vi "Build All.vi"() -> ()   [LabVIEW 2021]
uses:
  <vilib>/CIF Foundation/CIF LabVIEW Scripting/LV Scripting/Typedef/Version Increment.ctl
  <vilib>/CIF Foundation/CIF LabVIEW Scripting/LV Scripting/Typedef/Version.ctl
  <vilib>/CIF Foundation/CIF Core/CIFUtilities/Scripting/Build Libraries/LabVIEW Build Script/LabVIEW Build Script.lvclass/LabVIEW Build Script.ctl
  <vilib>/CIF Foundation/CIF LabVIEW Scripting/LV Scripting/SubVIs/Add Scripting Error.vi
  <vilib>/CIF Foundation/CIF Utilities/Errors/Append Error Location.vi
  <vilib>/AppBuilder/AB_API_Simple/Build (path).vi
  <vilib>/AppBuilder/AB_API_Simple/NI_App_Builder_API.lvlib
  <vilib>/CIF Foundation/CIF LabVIEW Scripting/LV Scripting/LV Scripting Utilities.lvlib
  <vilib>/CIF Foundation/CIF Core/CIFUtilities/Scripting/Build Libraries/LabVIEW Build Script/LabVIEW Build Script.lvclass
panel:
  out "error out 3":errorcluster
  out "error out 2":errorcluster
  out "Version":T1
  in  "String":string
  in  "Changes":string
  in  "Version Increment":T2
  out "error out":errorcluster
  out "Description":string
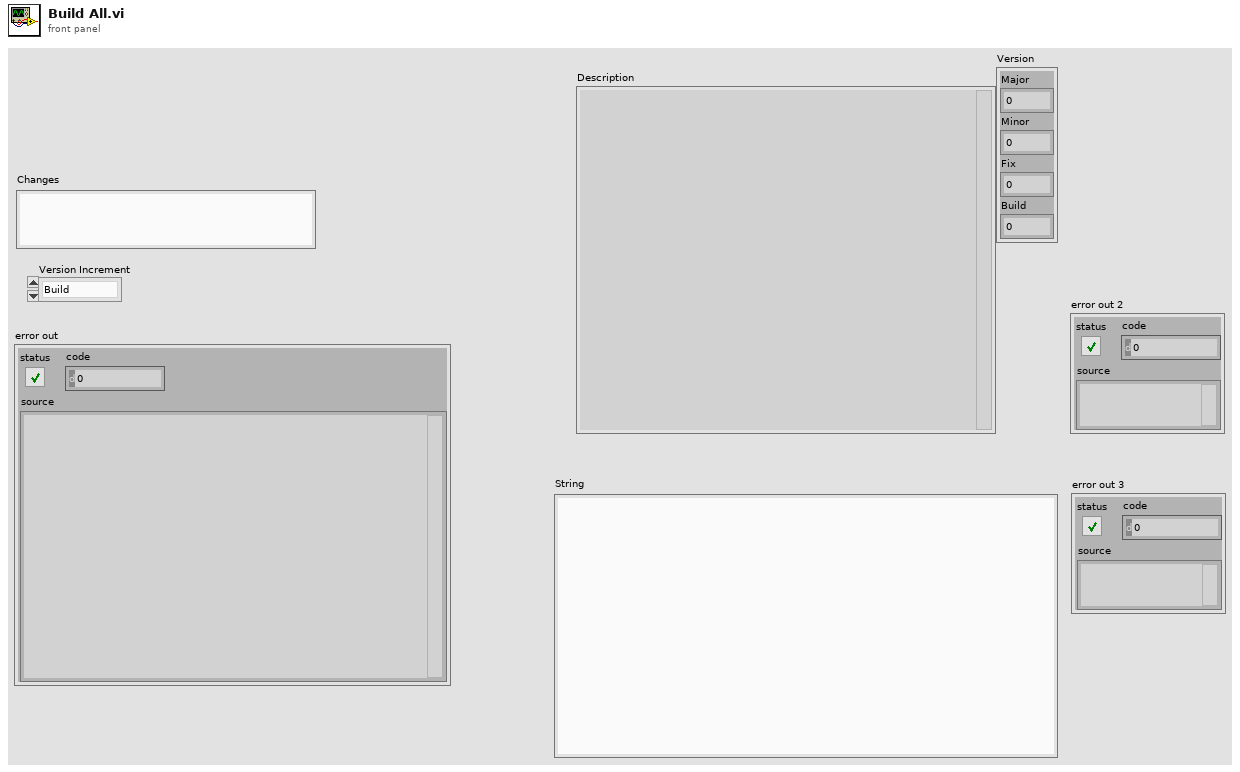
[diagram p1: front panel]
types:
  T1 = typedef "Version.ctl" = cluster{"Major":u16, "Minor":u16, "Fix":u16, "Build":u16}
  T2 = typedef "LV Scripting Utilities.lvlib/Version Increment.ctl" = enum16{"Build", "Fix", "Minor", "Major"}
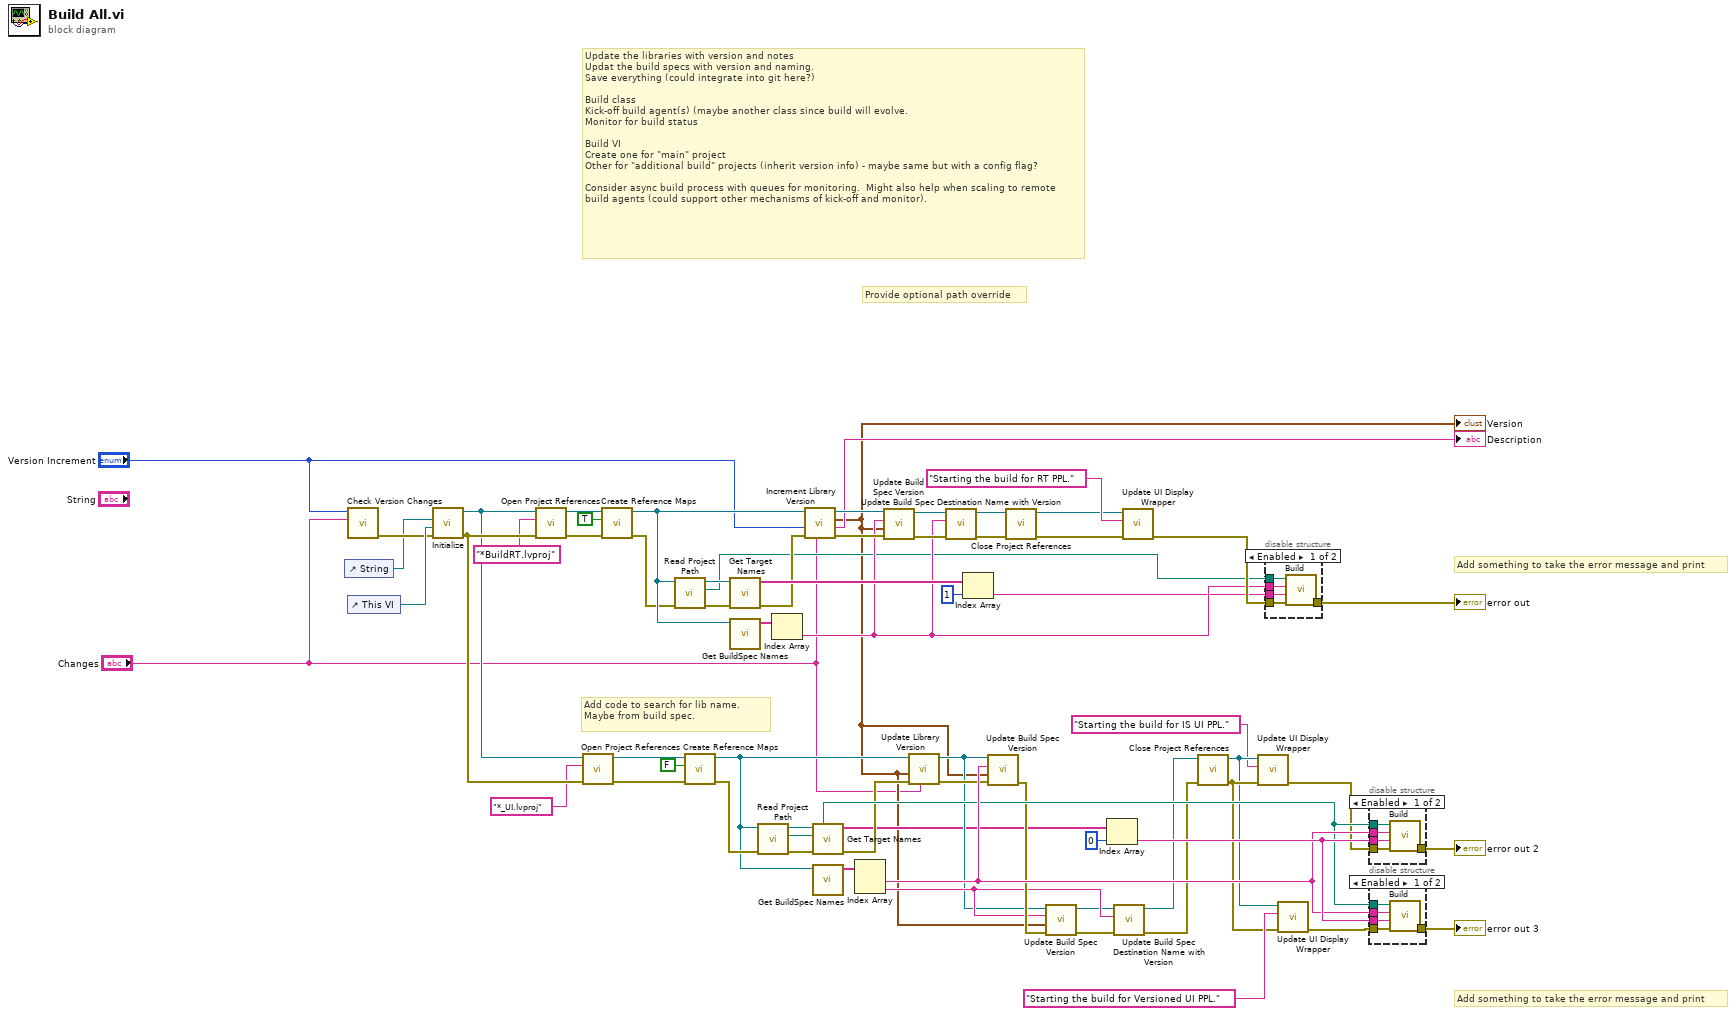
[diagram p0: block diagram]
diagram:
  # "Add code to search for lib name. Maybe from build spec."
  # "Add something to take the error message and print"
  # "Add something to take the error message and print"
  # "Update the libraries with version and notes\nUpdat the build specs with version and naming.\nSave everything (could integrate into git here?)\n\nBuild class\nKick-off build agent(s) (maybe another class since build will evolve.\nMonitor for build status\n\nBuild VI\nCreate one for \"main\" project\nOther for \"additional build\" projects (inherit version info) - maybe same but with a config flag?\n\nConsider async build process with queues for monitoring.  Might also help when scaling to remote build agents (could support other mechanisms of kick-off and monitor)."
  # "Provide optional path override"
  n1 = control-ref of="String"() -> (w12:refnum<vi>)
  n2 = call <vilib>:"Check Version Changes.vi"("Changes"="Changes", "Version Increment"="Version Increment") -> ("error out"=w17:errorcluster)  [unwired: 9 in]
  n3 = control-ref of="This VI"() -> (w24:refnum<vi>)
  n4 = call <vilib>:"Initialize.vi"("error in (no error)"=w17, "Calling VI"=w24, "UI Display"=w12) -> ("error out"=w38:errorcluster, "LabVIEW Build Script out"=w36:refnum<class "LabVIEW Build Script.lvclass">)  [unwired: 7 in]
  n5 = call <vilib>:"Open Project References.vi"("error in (no error)"=w38, "Search Pattern"="*BuildRT.lvproj" ("pattern"), "LabVIEW Build Script in"=w36) -> ("error out"=w15:errorcluster, "LabVIEW Build Script out"=w14:refnum<class "LabVIEW Build Script.lvclass">)  [unwired: 7 in]
  n6 = call <vilib>:"Open Project References.vi"("error in (no error)"=w38, "Search Pattern"="*_UI.lvproj" ("pattern"), "LabVIEW Build Script in"=w36) -> ("error out"=w50:errorcluster, "LabVIEW Build Script out"=w49:refnum<class "LabVIEW Build Script.lvclass">)  [unwired: 7 in]
  n7 = call <vilib>:"Create Reference Maps.vi"("error in (no error)"=w15, "RT Target"=TRUE, "LabVIEW Build Script in"=w14) -> ("error out"=w29:errorcluster, "LabVIEW Build Script out"=w30:refnum<class "LabVIEW Build Script.lvclass">)  [unwired: 7 in]
  n8 = call <vilib>:"Read Project Path.vi"("error in (no error)"=w29, "LabVIEW Build Script in"=w30) -> ("error out"=w31:errorcluster, "Project Path"=w8:path, "LabVIEW Build Script out"=w32:refnum<class "LabVIEW Build Script.lvclass">)  [unwired: 7 in]
  n9 = call <vilib>:"Create Reference Maps.vi"("error in (no error)"=w50, "RT Target"=FALSE, "LabVIEW Build Script in"=w49) -> ("error out"=w42:errorcluster, "LabVIEW Build Script out"=w41:refnum<class "LabVIEW Build Script.lvclass">)  [unwired: 7 in]
  n10 = call <vilib>:"Get Target Names.vi"("error in (no error)"=w31, "LabVIEW Build Script in"=w32) -> ("error out"=w25:errorcluster, "Project Targets"=w27:string[])  [unwired: 8 in]
  n11 = call <vilib>:"Get BuildSpec Names.vi"("LabVIEW Build Script in"=w30) -> ("BuildSpecs"=w26:string[])  [unwired: 10 in]
  n12 = call <vilib>:"Read Project Path.vi"("error in (no error)"=w42, "LabVIEW Build Script in"=w41) -> ("error out"=w40:errorcluster, "Project Path"=w64:path, "LabVIEW Build Script out"=w39:refnum<class "LabVIEW Build Script.lvclass">)  [unwired: 7 in]
  n13 = Index Array(array=w26) -> (element=w10:string)  [unwired: 1 in]
  n14 = call <vilib>:"Increment Library Version.vi"("Changes"="Changes", "error in (no error)"=w25, "Version Increment"="Version Increment", "LabVIEW Build Script in"=w30) -> ("error out"=w19:errorcluster, "Description"=→"Description":string, "Version"=w3:T1, "LabVIEW Build Script out"=w18:refnum<class "LabVIEW Build Script.lvclass">)  [unwired: 4 in]
  "Version" <- w3
  n15 = call <vilib>:"Get Target Names.vi"("error in (no error)"=w40, "LabVIEW Build Script in"=w39) -> ("error out"=w46:errorcluster, "Project Targets"=w44:string[])  [unwired: 8 in]
  n16 = call <vilib>:"Get BuildSpec Names.vi"("LabVIEW Build Script in"=w41) -> ("BuildSpecs"=w45:string[])  [unwired: 10 in]
  n17 = Index Array(array=w45) -> (element #1=w65:string, element #2=w55:string)  [unwired: 2 in]
  n18 = call <vilib>:"Update Build Spec Version.vi"("error in (no error)"=w19, "Version"=w3, "Search Pattern"=w10, "LabVIEW Build Script in"=w18) -> ("error out"=w21:errorcluster, "LabVIEW Build Script out"=w20:refnum<class "LabVIEW Build Script.lvclass">)  [unwired: 6 in]
  n19 = call <vilib>:"Update Library Version.vi"("Changes"="Changes", "error in (no error)"=w46, "Version"=w3, "LabVIEW Build Script in"=w41) -> ("error out"=w53:errorcluster, "LabVIEW Build Script out"=w52:refnum<class "LabVIEW Build Script.lvclass">)  [unwired: 5 in, 1 out]
  n20 = call <vilib>:"Update Build Spec Destination Name with Version.vi"("error in (no error)"=w21, "Search Pattern"=w10, "LabVIEW Build Script in"=w20) -> ("error out"=w23:errorcluster, "LabVIEW Build Script out"=w22:refnum<class "LabVIEW Build Script.lvclass">)  [unwired: 7 in]
  n21 = Index Array(array=w27, index=1) -> (element=w9:string)
  n22 = call <vilib>:"Update Build Spec Version.vi"("error in (no error)"=w53, "Version"=w3, "Search Pattern"=w65, "LabVIEW Build Script in"=w52) -> ("error out"=w56:errorcluster)  [unwired: 6 in, 1 out]
  n23 = call <vilib>:"Close Project References.vi"("error in (no error)"=w23, "LabVIEW Build Script in"=w22) -> ("error out"=w34:errorcluster, "LabVIEW Build Script out"=w33:refnum<class "LabVIEW Build Script.lvclass">)  [unwired: 8 in]
  n24 = call <vilib>:"Update Build Spec Version.vi"("error in (no error)"=w56, "Version"=w3, "Search Pattern"=w55, "LabVIEW Build Script in"=w52) -> ("error out"=w54:errorcluster, "LabVIEW Build Script out"=w51:refnum<class "LabVIEW Build Script.lvclass">)  [unwired: 6 in]
  n25 = Index Array(array=w44, index=0) -> (element=w66:string)
  n26 = call <vilib>:"Update Build Spec Destination Name with Version.vi"("error in (no error)"=w54, "Search Pattern"=w55, "LabVIEW Build Script in"=w51) -> ("error out"=w58:errorcluster, "LabVIEW Build Script out"=w57:refnum<class "LabVIEW Build Script.lvclass">)  [unwired: 7 in]
  n27 = call <vilib>:"Update UI Display Wrapper.vi"("error in (no error)"=w34, "Update for Display"="Starting the build for RT PPL.", "LabVIEW Build Script in"=w33) -> ("error out"=w11:errorcluster)  [unwired: 8 in]
  n28 = call <vilib>:"Close Project References.vi"("error in (no error)"=w58, "LabVIEW Build Script in"=w57) -> ("error out"=w61:errorcluster, "LabVIEW Build Script out"=w60:refnum<class "LabVIEW Build Script.lvclass">)  [unwired: 8 in]
  n29 = call <vilib>:"Update UI Display Wrapper.vi"("error in (no error)"=w61, "Update for Display"="Starting the build for IS UI PPL.", "LabVIEW Build Script in"=w60) -> ("error out"=w48:errorcluster)  [unwired: 8 in]
  n30 = disable-structure shown="Enabled" {
    disable-tunnel: w8 -> [w71 _]
    disable-tunnel: w9 -> [w70 _]
    disable-tunnel: w10 -> [w69 _]
    disable-tunnel: w11 -> [w68 w72]
    disable-tunnel: [w67 w72] -> w5
    frame Enabled {
      n31 = call-poly <vilib>:"Build.vi"("error in (no error)"=w68, "Name of target (My Computer)"=w70, "Name of build specification (if empty: build all)"=w69, "Path to project"=w71) -> ("error out"=w67:errorcluster)  [unwired: 6 in, 1 out]
    }
    frame Disabled {
    }
  }
  "error out" <- w5
  n32 = call <vilib>:"Update UI Display Wrapper.vi"("error in (no error)"=w61, "Update for Display"="Starting the build for Versioned UI PPL.", "LabVIEW Build Script in"=w60) -> ("error out"=w63:errorcluster)  [unwired: 8 in]
  n33 = disable-structure shown="Enabled" {
    disable-tunnel: w64 -> [w77 _]
    disable-tunnel: w66 -> [w76 _]
    disable-tunnel: w65 -> [w75 _]
    disable-tunnel: w48 -> [w74 w78]
    disable-tunnel: [w73 w78] -> w6
    frame Enabled {
      n34 = call-poly <vilib>:"Build.vi"("error in (no error)"=w74, "Name of target (My Computer)"=w76, "Name of build specification (if empty: build all)"=w75, "Path to project"=w77) -> ("error out"=w73:errorcluster)  [unwired: 6 in, 1 out]
    }
    frame Disabled {
    }
  }
  "error out 2" <- w6
  n35 = disable-structure shown="Enabled" {
    disable-tunnel: w64 -> [w83 _]
    disable-tunnel: w66 -> [w82 _]
    disable-tunnel: w65 -> [w81 _]
    disable-tunnel: w63 -> [w80 w84]
    disable-tunnel: [w79 w84] -> w7
    frame Enabled {
      n36 = call-poly <vilib>:"Build.vi"("error in (no error)"=w80, "Name of target (My Computer)"=w82, "Name of build specification (if empty: build all)"=w81, "Path to project"=w83) -> ("error out"=w79:errorcluster)  [unwired: 6 in, 1 out]
    }
    frame Disabled {
    }
  }
  "error out 3" <- w7
